vi "Write FPGA VI Reference Out.vi"(8 "error in (no error)":errorcluster, 10 "FPGA Interface":T1, 11 "FPGASession in":refnum<class "FPGASession.lvclass">) -> (0 "error out":errorcluster, 3 "FPGASession out":refnum<class "FPGASession.lvclass">)   [LabVIEW 2013, in "FPGASession.lvclass"]
uses:
  FPGASession.lvclass
  RT/FPGASession/FPGARef.ctl
  FPGASession.lvclass/FPGASession.ctl
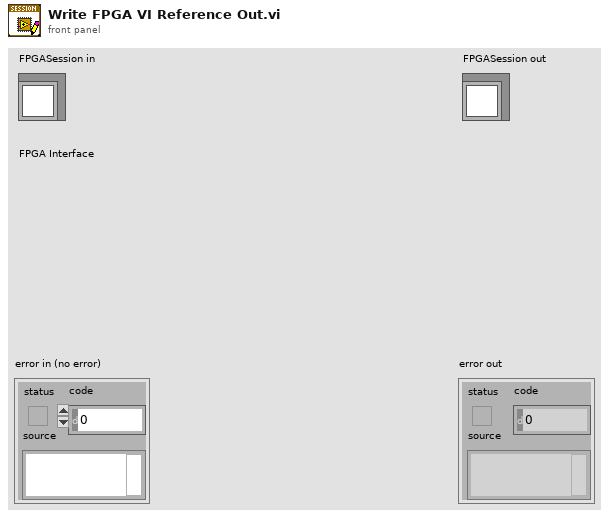
[diagram p1: front panel]
types:
  T1 = typedef "FPGASession.lvclass/FPGARef.ctl" = refnum<k20>
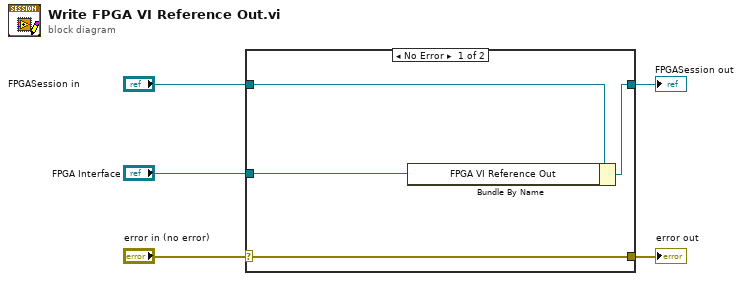
[diagram p0: block diagram]
diagram:
  n1 = case shown="No Error" "error in (no error)" {
    selector: "error in (no error)" -> [w9 w10]
    tunnel: [w9 w10] -> w4
    tunnel: [w7 w11] -> w2
    tunnel: "FPGASession in" -> [w8 w11]
    tunnel: "FPGA Interface" -> [w6 _]
    frame No Error {
      n2 = Bundle By Name(cluster=w8, "FPGA VI Reference Out"=w6) -> (w7:refnum<class "FPGASession.lvclass">)
    }
    frame Error {
    }
  }
  "error out" <- w4
  "FPGASession out" <- w2
